vi "XLP80_Action_InitWriteB_Preconditions.vi"(8 "err in":errorcluster) -> (0 "err out":errorcluster)   [LabVIEW 2021]
uses:
  XLP80_Globals/Globals_Settings_XLP80.vi
  XLP80_Globals/XLP80_CAN_Globals.vi
  XLP80_Globals/XLP80_Globals_Referenzen.vi
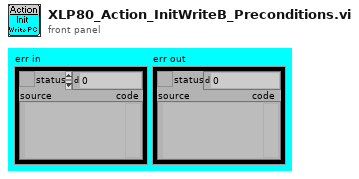
[diagram p1: front panel]
types:
  T1 = cluster{"Signal Name":string[], "Description":string[], "Unit":string[], "Default":dbl[], "Min":dbl[], "Max":dbl[], "Preconditions":bool[], "HV & Software":bool[], "Basis Funktion":bool[], "Power Management":bool[], "OperationMode":bool[], "Shutdown":bool[], "Alarm":bool[], "LogEnable":bool[]}
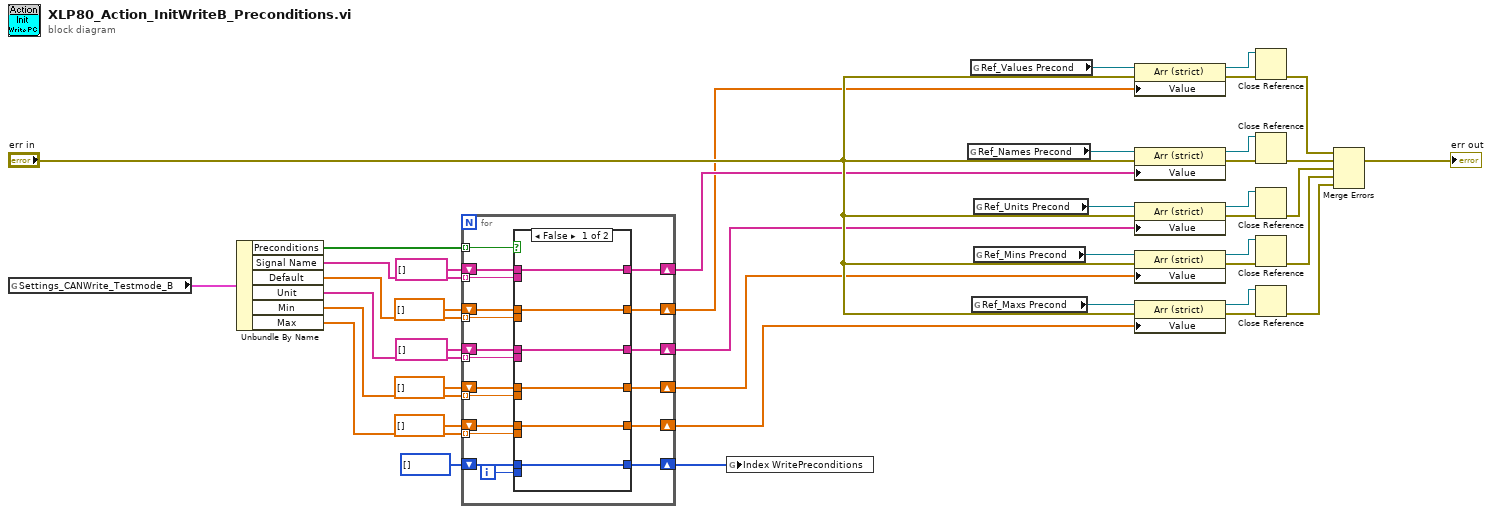
[diagram p0: block diagram]
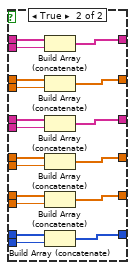
[diagram p2: hidden frame]
diagram:
  n1 = global read "Globals_Settings_XLP80.vi" "Settings_CANWrite_Testmode_B"() -> (w41:T1)
  n2 = Unbundle By Name(w41) -> ("Preconditions"=w30:bool[], "Signal Name"=w33:string[], "Default"=w23:dbl[], "Unit"=w18:string[], "Min"=w17:dbl[], "Max"=w16:dbl[])
  n3 = for {
    tunnel: w30 -> [w60] mode=indexing
    shift-right: [w57] -> w29
    shift-left: string[] [] ("Signal Name") -> [w59]
    shift-right: [w54] -> w31
    shift-left: i32[] [] -> [w56]
    tunnel: w33 -> [w58] mode=indexing
    shift-right: [w51] -> w22
    shift-left: dbl[] [] ("Default") -> [w53]
    tunnel: w23 -> [w52] mode=indexing
    shift-right: [w50] -> w2
    shift-left: dbl[] [] ("Default") -> [w48]
    tunnel: w17 -> [w49] mode=indexing
    shift-right: [w45] -> w1
    shift-left: dbl[] [] ("Default") -> [w47]
    tunnel: w16 -> [w46] mode=indexing
    shift-right: [w44] -> w3
    shift-left: string[] [] ("Signal Name") -> [w42]
    tunnel: w18 -> [w43] mode=indexing
    i -> [w55]
    n4 = case shown="False" w60 {
      tunnel: w59 -> [w66 w84]
      tunnel: w58 -> [_ w83]
      tunnel: [w66 w82] -> w57
      tunnel: w56 -> [w65 w81]
      tunnel: w55 -> [_ w80]
      tunnel: [w65 w79] -> w54
      tunnel: w53 -> [w64 w78]
      tunnel: w52 -> [_ w77]
      tunnel: [w64 w76] -> w51
      tunnel: w48 -> [w62 w73]
      tunnel: w49 -> [_ w74]
      tunnel: [w62 w75] -> w50
      tunnel: w47 -> [w61 w72]
      tunnel: w46 -> [_ w71]
      tunnel: [w61 w70] -> w45
      tunnel: w42 -> [w63 w67]
      tunnel: w43 -> [_ w68]
      tunnel: [w63 w69] -> w44
      frame False {
      }
      frame True {
        n5 = Build Array (concatenate)(w84, w83) -> (w82:string[])
        n6 = Build Array (concatenate)(w78, w77) -> (w76:dbl[])
        n7 = Build Array (concatenate)(w67, w68) -> (w69:string[])
        n8 = Build Array (concatenate)(w73, w74) -> (w75:dbl[])
        n9 = Build Array (concatenate)(w72, w71) -> (w70:dbl[])
        n10 = Build Array (concatenate)(w81, w80) -> (w79:i32[])
      }
    }
  }
  n11 = global write "XLP80_CAN_Globals.vi" "Index WritePreconditions"(w31) -> ()
  n12 = global read "XLP80_Globals_Referenzen.vi" "Ref_Names Precond"() -> (w36:refnum<vi>)
  n13 = global read "XLP80_Globals_Referenzen.vi" "Ref_Values Precond"() -> (w26:refnum<vi>)
  n14 = global read "XLP80_Globals_Referenzen.vi" "Ref_Maxs Precond"() -> (w7:refnum<vi>)
  n15 = global read "XLP80_Globals_Referenzen.vi" "Ref_Units Precond"() -> (w15:refnum<vi>)
  n16 = global read "XLP80_Globals_Referenzen.vi" "Ref_Mins Precond"() -> (w12:refnum<vi>)
  n17 = property class="Arr (strict)"(reference=w26, error in="err in", "Value"=w22) -> (reference out=w28:refnum<vi>, error out=w27:errorcluster)
  n18 = property class="Arr (strict)"(reference=w36, error in="err in", "Value"=w29) -> (reference out=w37:refnum<vi>, error out=w38:errorcluster)
  n19 = property class="Arr (strict)"(reference=w15, error in="err in", "Value"=w3) -> (reference out=w13:refnum<vi>, error out=w14:errorcluster)
  n20 = property class="Arr (strict)"(reference=w12, error in="err in", "Value"=w2) -> (reference out=w11:refnum<vi>, error out=w10:errorcluster)
  n21 = property class="Arr (strict)"(reference=w7, error in="err in", "Value"=w1) -> (reference out=w8:refnum<vi>, error out=w9:errorcluster)
  n22 = Close Reference(reference=w28, error in (no error)=w27) -> (error out=w25:errorcluster)
  n23 = Close Reference(reference=w37, error in (no error)=w38) -> (error out=w35:errorcluster)
  n24 = Close Reference(reference=w13, error in (no error)=w14) -> (error out=w6:errorcluster)
  n25 = Close Reference(reference=w11, error in (no error)=w10) -> (error out=w5:errorcluster)
  n26 = Close Reference(reference=w8, error in (no error)=w9) -> (error out=w4:errorcluster)
  n27 = Merge Errors(w25, w35, w6, w5, w4) -> (→"err out":errorcluster)
